vi "Function.vi"(8 "error in (no error)":errorcluster, 9 "Numeric B":i32, 10 "Numeric A":i32, 11 "Two Terminal in":refnum<class "Less Equal_I32.lvclass">) -> (0 "error out":errorcluster, 2 "Result":bool, 3 "Two Terminal out":refnum<class "Less Equal_I32.lvclass">)   [LabVIEW 2021, in "Less Equal_I32.lvclass"]
uses:
  Less Equal_I32.lvclass
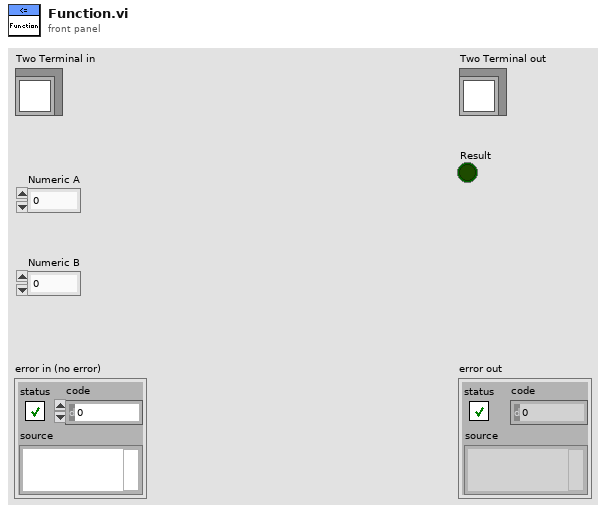
[diagram p1: front panel]
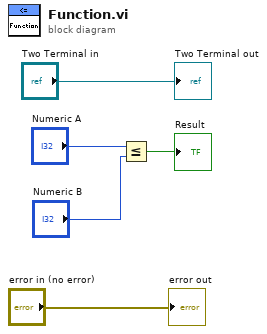
[diagram p0: block diagram]
diagram:
  n1 = Less Or Equal?(x="Numeric A", y="Numeric B") -> (x <= y?=→"Result":bool)
  "error out" <- "error in (no error)"
  "Two Terminal out" <- "Two Terminal in"
